vi "Convert Bool Fails to Strings.vi"(1 "Possible Failure Modes":bool[](array[boolean])) -> (0 "String":string)   [LabVIEW 2011]
uses:
  OpenG SearchArray/Search 1D Array (Boolean)__ogtk.vi
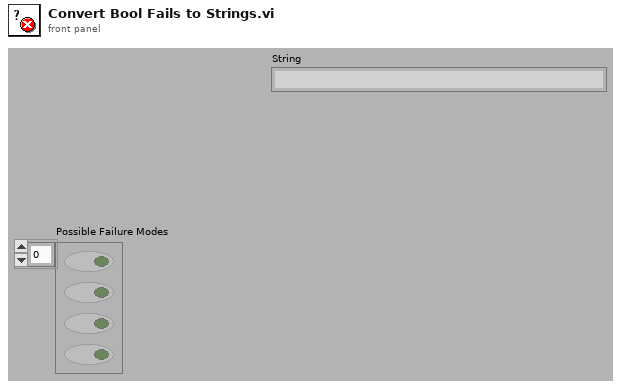
[diagram p1: front panel]
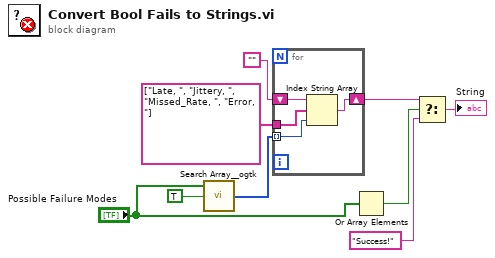
[diagram p0: block diagram]
diagram:
  n1 = call-poly "Search Array__ogtk.vi"("Array"="Possible Failure Modes", "Element Data"=TRUE) -> ("Indices of Elements"=w4:i32[])  [unwired: 7 in]
  n2 = for {
    tunnel: w4 -> [w13] mode=indexing
    tunnel: string[] ["Late, ", "Jittery, ", "Missed_Rate, ", "Error, "] -> [w12]
    shift-right: [w11] -> w1
    shift-left: "" -> [w10]
    n3 = Index String Array(1:w13, 2:w12, 3:w10) -> (0:w11:string)
  }
  n4 = Or Array Elements(Boolean array="Possible Failure Modes") -> (logical OR=w9:bool)
  n5 = Select(t=w1, s=w9, f="Success!") -> (s? t:f=→"String":string)
